vi "Project Data InitialS4.vi"(11 "configuration file path":path=path "C:/Users/MyUser/Desktop/新文字文件 - 複製.txt") -> (1 "Step Content":string[][](table), 2 "Retry":i32, 3 "process cluster":cluster{string[], i32[]})   [LabVIEW 2019]
uses:
  <vilib>/Utility/config.llb/Read Key (String).vi
  <vilib>/Utility/config.llb/NI_LVConfig.lvlib
  Ctrl/StationCmdSelect.ctl
  FlowCtrl Class/LineScan/LineScan.lvclass
  Ctrl/MeasureDisplayTab.ctl
  LLB/Commonly VI/Main Glb.vi
  LLB/Commonly VI.lvlib
  Ctrl/Table Save.ctl
  Ctrl/Auto Inspection Station Name2.ctl
  Ctrl/Auto Inspection Data Name.ctl
  Ctrl/S2 Station IO.ctl
panel:
  out "S2 receive":string
  out "Blue Scan2 receive":string
  out "T2 buffer":string
  out "T2 μA":dbl format="%#_6f"
  out "T1 buffer":string
  out "T1 μA":dbl format="%#_6f"
  in  "error in (no error)":errorcluster
  out "Blue Scan receive":string
  out "S1 receive":string
  out "Program receive":string
  out "Initial receive":string
  out "Act Step":i32
  out "retry次數":string[](array[string])
  in  "stop":bool
  out "Boolean":bool=TRUE
  in  "Numeric 3":i32
  out "format receive":string
  out "CurrentCmd":string
  out "Numeric":dbl
  out "LOG":string[][](array[string])
  in  "Enum":T1(ring)=enum."Add"
  in  "Table Control 3":string[][](table)=[["PCBA BARCODE", ""], ["硬體(Tool初始化)", ""], ["company(Tool初始化)", ""], ["耗電流 uA(電流表)", "T"], ["電池負載電壓", "T"], ["晶片ID(Tool FORMAT)", "F"], ["雷雕ID(TOOl scan、藍芽接收器)", "S"], ["Format(Tool FORMAT)", "F"], ["Programe(Tool Programe)", "P"]]
  in  "SN":string
  out "Array 3":cluster{"Table Control":string[][]}[](array[cluster])
  in  "Table Control":string[][](table)=[["PCBA BARCODE", ""], ["硬體(Tool初始化)", ""], ["company(Tool初始化)", ""], ["耗電流 uA(電流表)", "T"], ["電池負載電壓", "T"], ["晶片ID(Tool FORMAT)", "F"], ["雷雕ID(TOOl scan、藍芽接收器)", "S"], ["Format(Tool FORMAT)", "F"], ["Programe(Tool Programe)", "P"]]
  out "subarray":string[](array[string])
  out "array":string[](array[string])
  out "Process":string[](array[string])
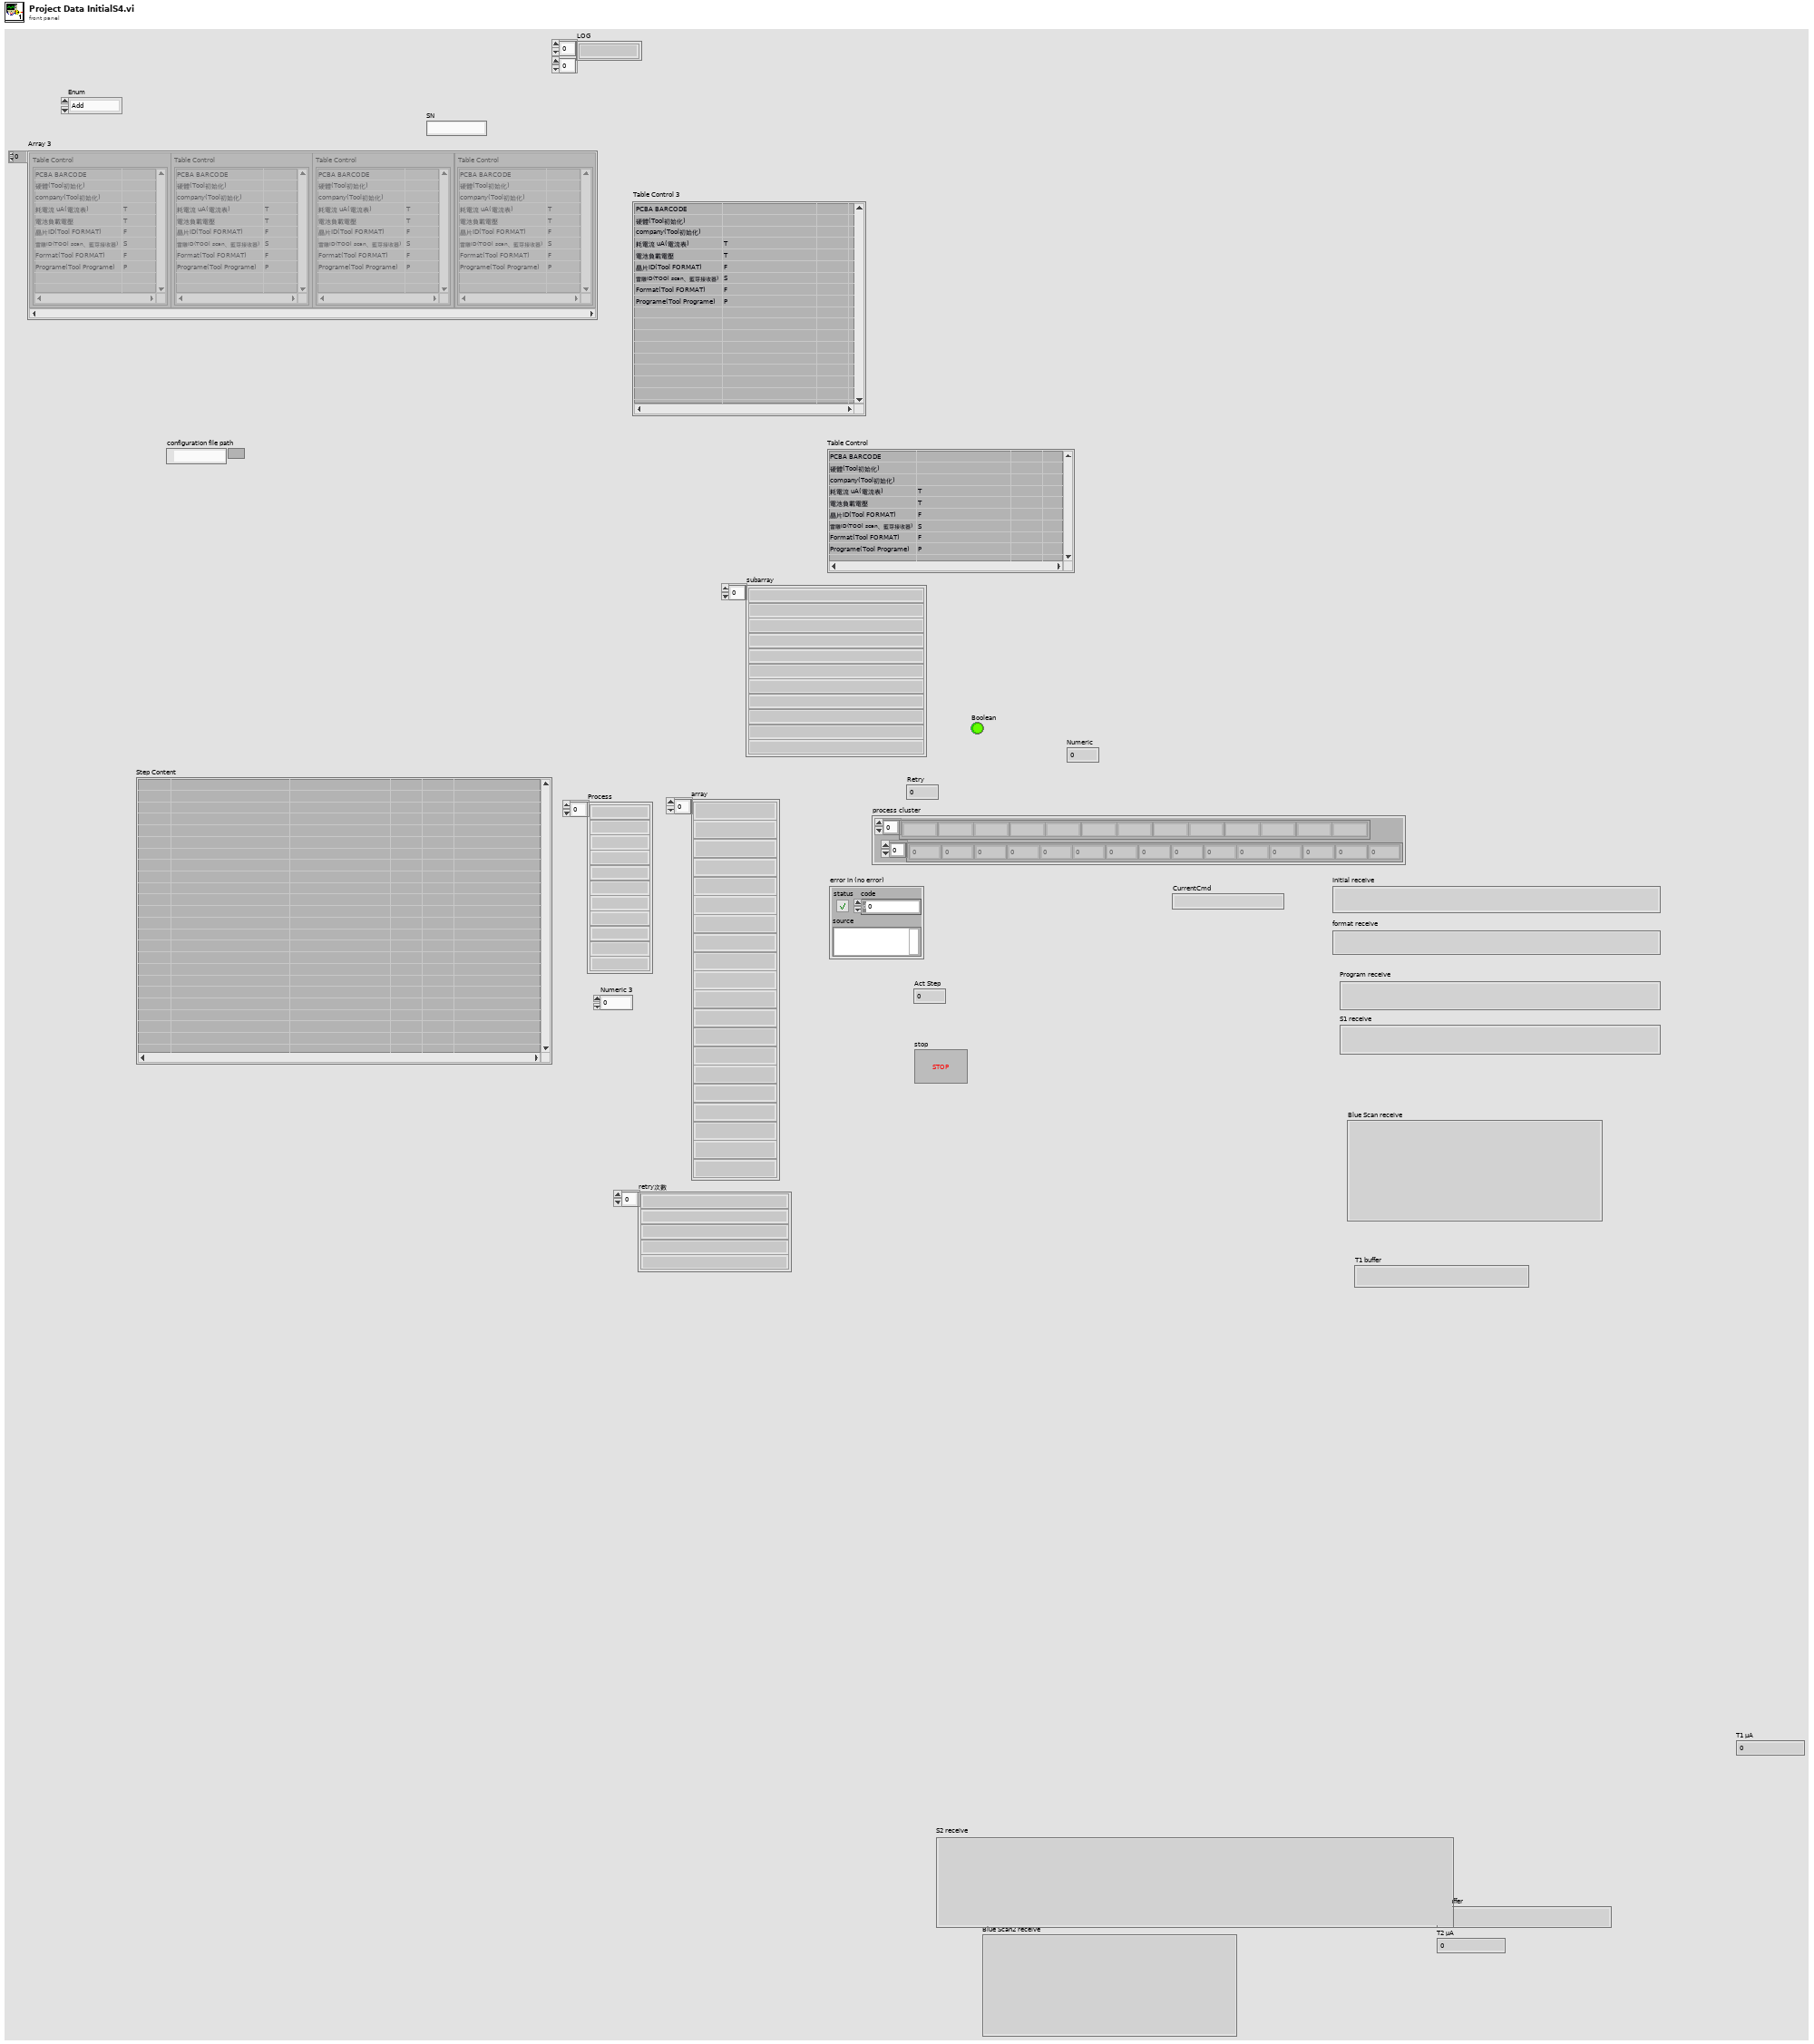
[diagram p1: front panel]
types:
  T1 = enum16{"initial", "Add", "Write", "Replace", "Delete", "REad"}
  T2 = typedef "NI_LVConfig.lvlib/Config Data RefNum.ctl" = refnum<k1>
  T3 = typedef "StationCmdSelect.ctl" = enum16{"Action", "Command", "Return", "DTime", "Retry"}
  T4 = typedef "Auto Inspection Data Name.ctl" = enum16{"LocalRun", "ItemSN(TimeCode)", "CurrentAction", "Error", "Data", "OKNG", "電壓值", "電壓值判斷", "電流值", "電流值判斷", "Laser1 Data", "Laser2 Data", "Laser OKNG", "StationNO"}
  T5 = typedef "Auto Inspection Station Name2.ctl" = enum16{"S1Barcode", "S2Measure", "S3Measure", "S4Measure", "S5Measure", "S11_LaserCheck", "S8_Vision AI"}
  T6 = typedef "Table Save.ctl" = enum16{"initial", "Add", "Write", "Replace", "Delete", "REad", "RedTable", "Load"}
  T7 = typedef "MeasureDisplayTab.ctl" = enum16{"Tray Barcode", "PCBA BARCODE", "硬體(Tool初始化)", "company(Tool初始化)", "耗電流 uA(電流表)", "電池負載電壓", "晶片ID(Tool FORMAT)", "雷雕ID(TOOl scan、藍芽接收器)", "Format(Tool FORMAT)", "Programe(Tool Programe)", "MAC(藍芽接收器)", "ID(藍芽接收器)", "KPA(藍芽接收器)", "溫度(藍芽接收器)", "SENSOR電池電壓(藍芽接收器)", "RSSI(藍芽接收器)", "SensorType_315(FSK scan)", "FSKsnVol_315(FSK scan)", "FSKscanl_315(FSK scan)", "P_315(FSK scan)", "T_315(FSK scan)", "SensorType_433(ASK scan)", "ASKsnVol_433(ASK scan)", "ASKscan_433(ASK scan)", "P_433(ASK scan)", "T_433(ASK scan)", "測高Data"}
  T8 = typedef "S2 Station IO.ctl" = enum16{"S2站PC動作中_20", "電流量測完成產品OK_21", "電流量測完成產品NG_22", "S2站Format 執行_23", "S2 Format OK_24", "S2 Format NG_25", "S2站燒入執行_26", "S2站燒入OK_27", "S2站燒入NG_28", "S2站動作完成_29", "S3 PC動作中_30", "S3 Format 此站執行_31", "S3 Format OK_32", "S3 Format NG_33", "S3 燒入程式 此站執行_34", "S3 燒入程式 OK_35", "S3 燒入程式 NG_36", "S3 備用_37", "S3 備用_38", "S3 動作完成_39", "S4 PC動作中_40", "S4 量測完成 產品正常_41", "S4 量測完成 產品NG_42", "S4 Format 此站執行_43", "S4 Format OK_44", "S4 Format NG_45", "S4 燒入 此站不執行_46", "S4 燒入程式 OK_47", "S4 燒入程式 NG_48", "S4 藍芽Scan OK_49", "S4 藍芽Scan NG_50", "S4 動作完成_51", "給PLC要量電流訊號", "給PLC要量電壓訊號"}
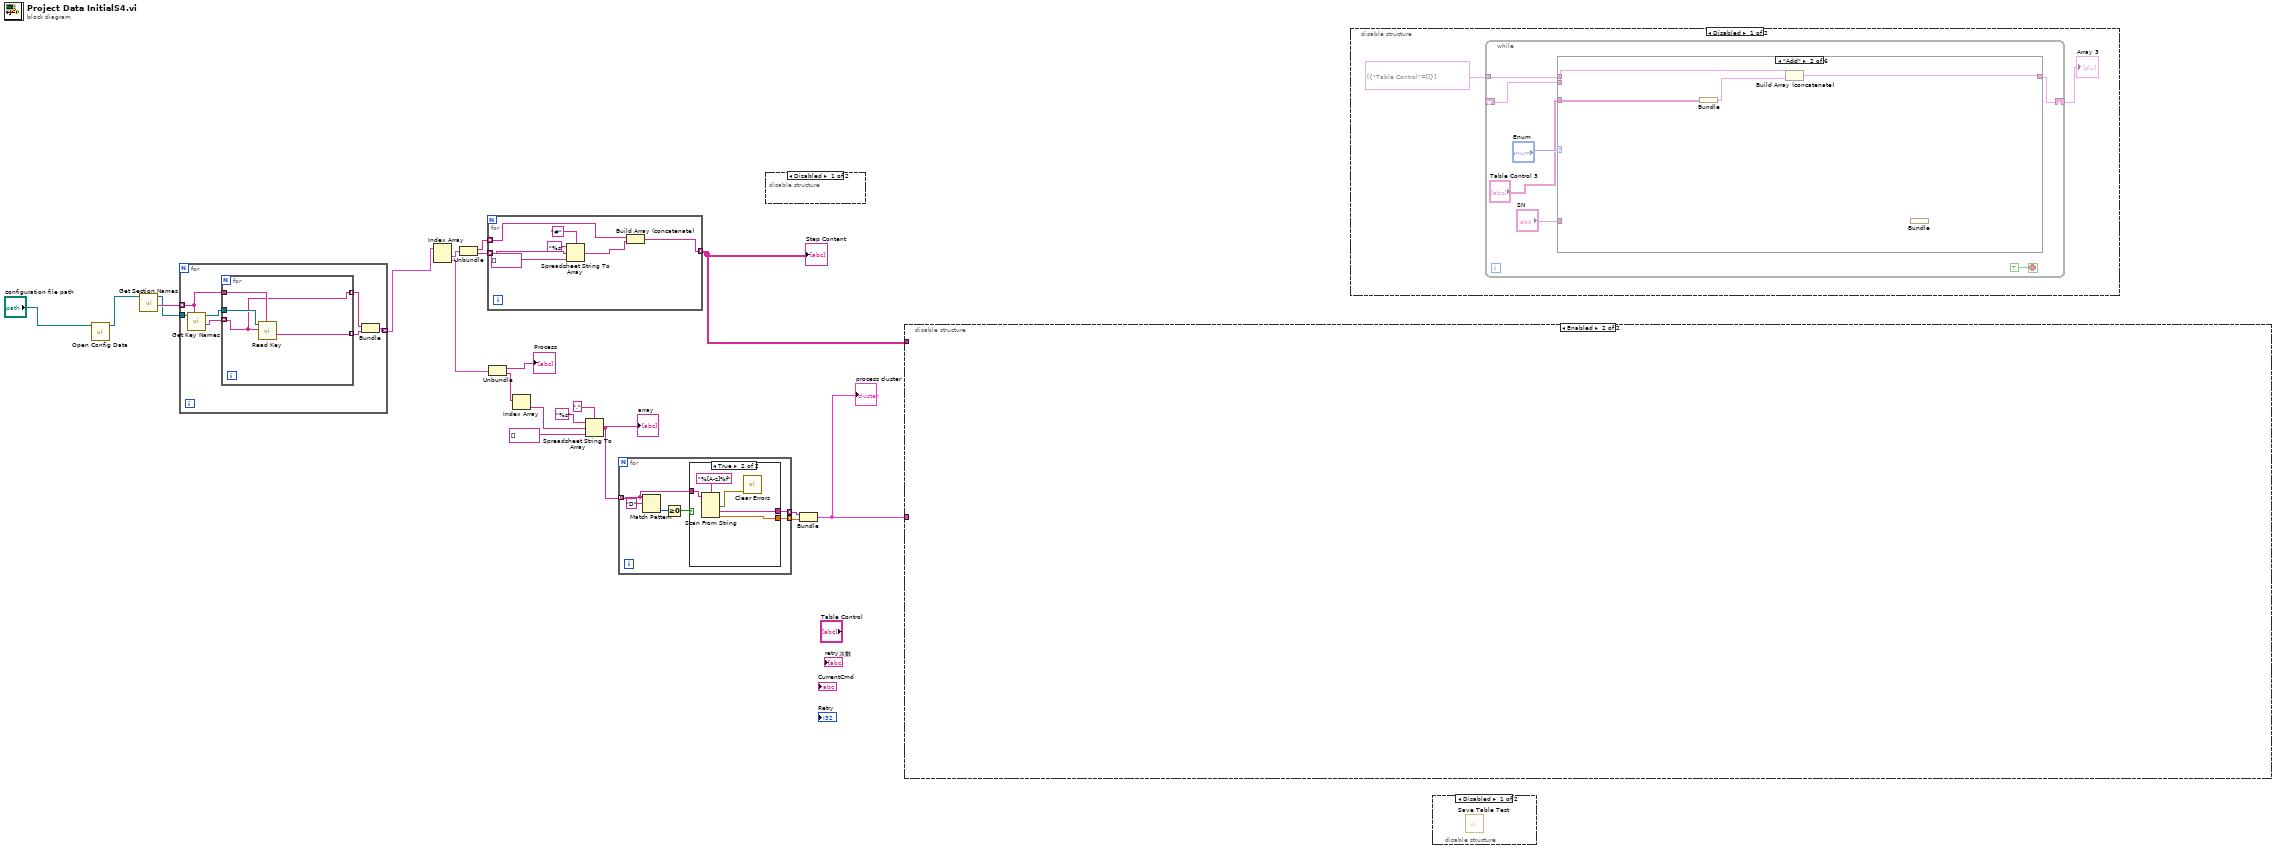
[diagram p0: block diagram]
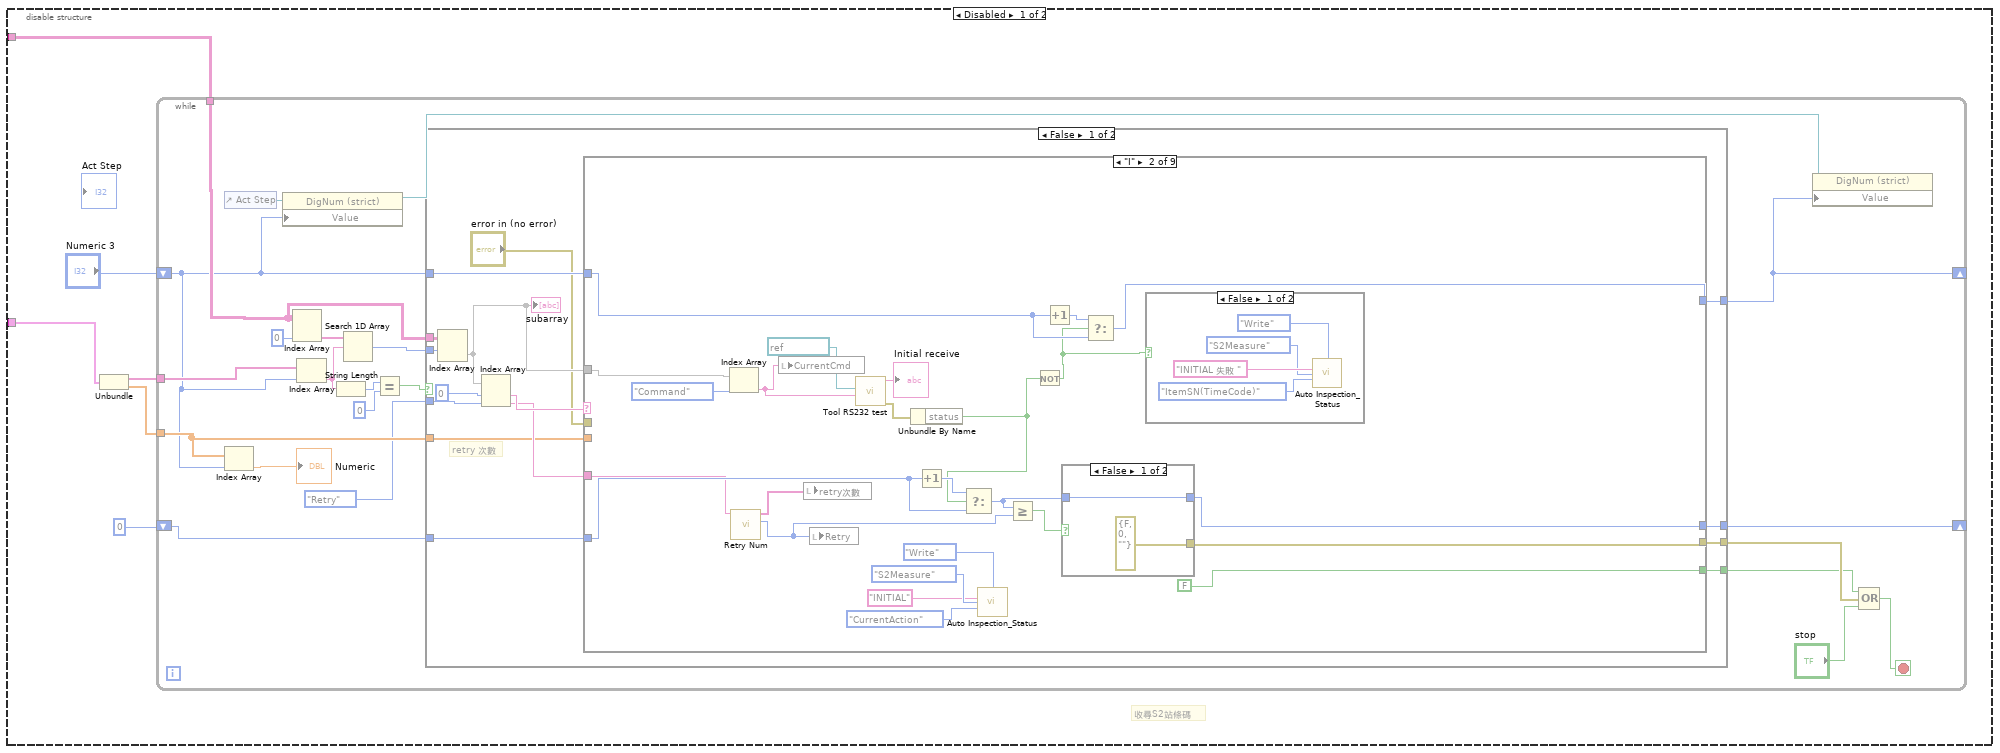
[diagram p3: hidden frame]
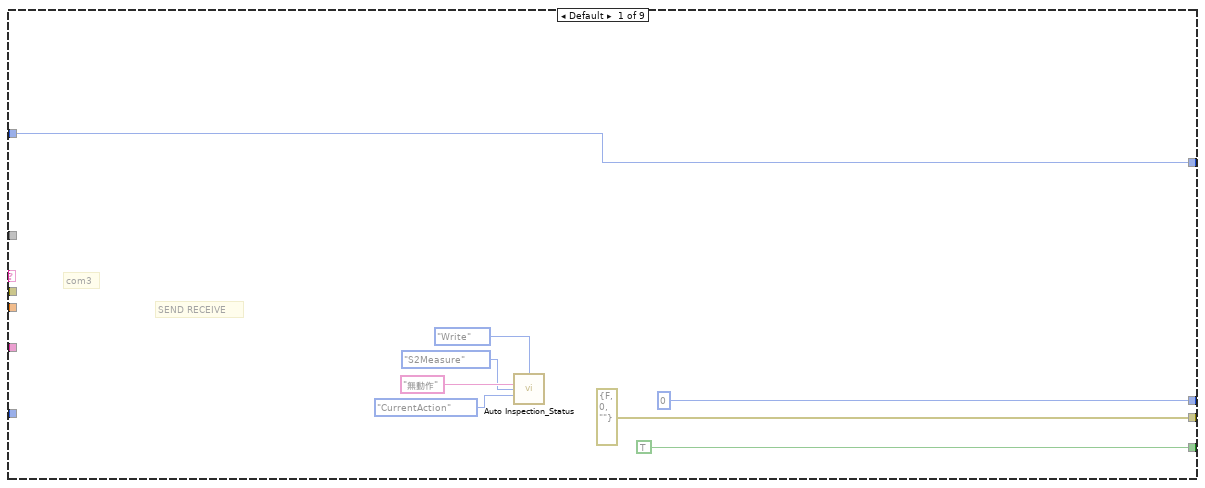
[diagram p4: hidden frame]
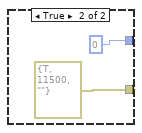
[diagram p6: hidden frame]
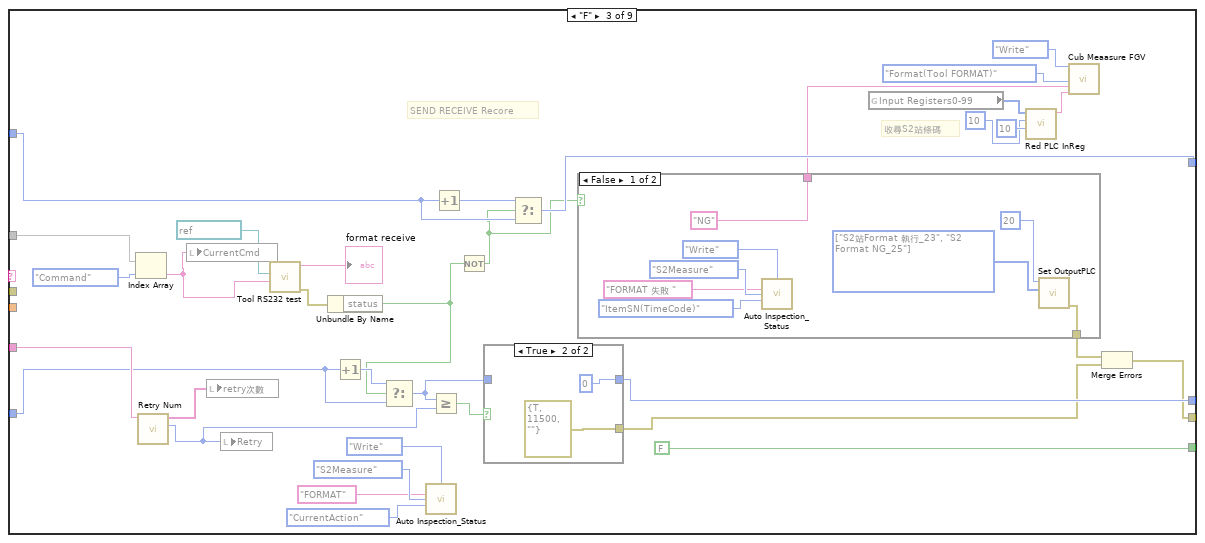
[diagram p7: hidden frame]
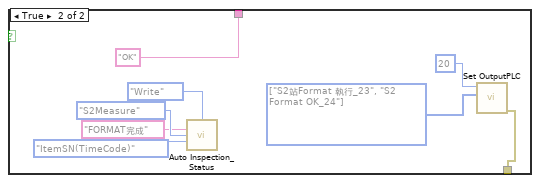
[diagram p8: hidden frame]
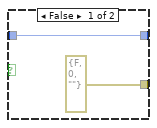
[diagram p9: hidden frame]
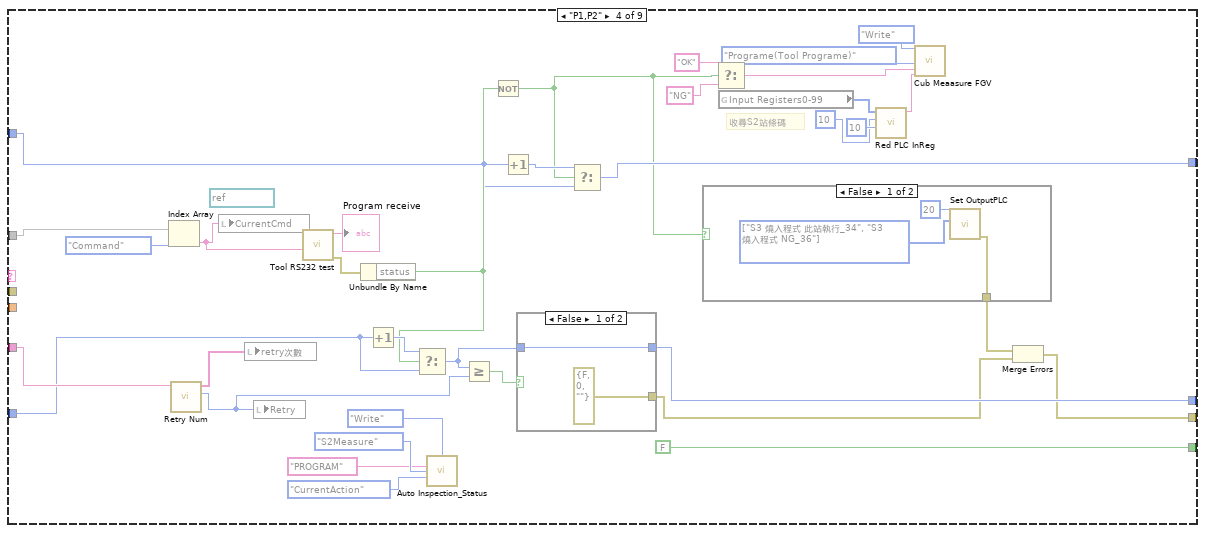
[diagram p10: hidden frame]
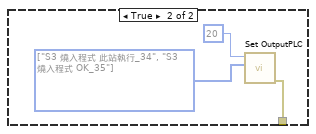
[diagram p11: hidden frame]
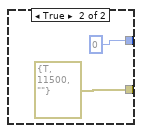
[diagram p12: hidden frame]
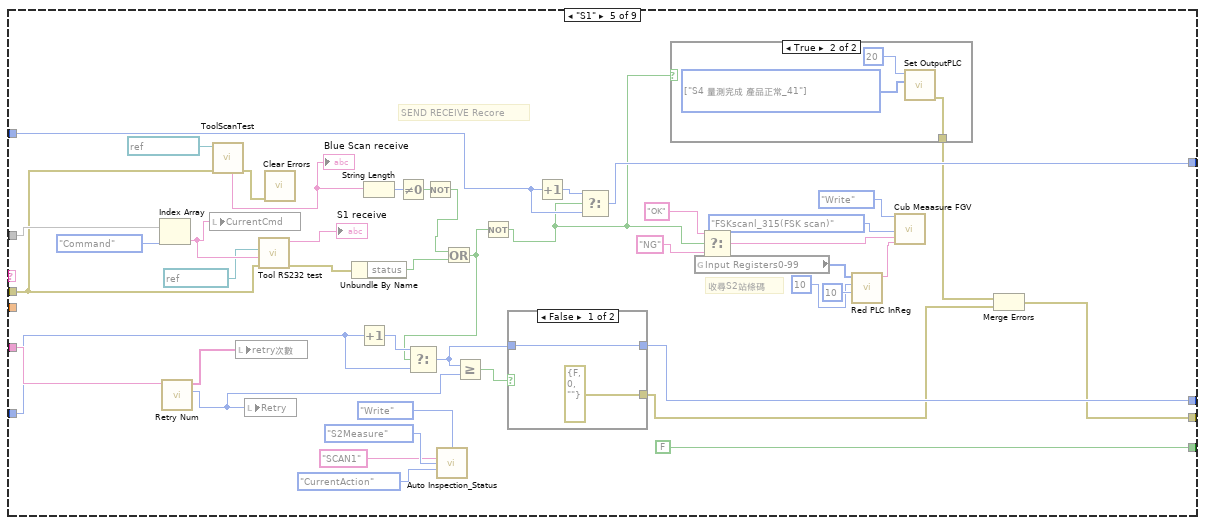
[diagram p13: hidden frame]
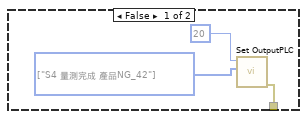
[diagram p14: hidden frame]
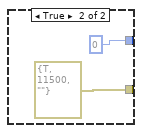
[diagram p15: hidden frame]
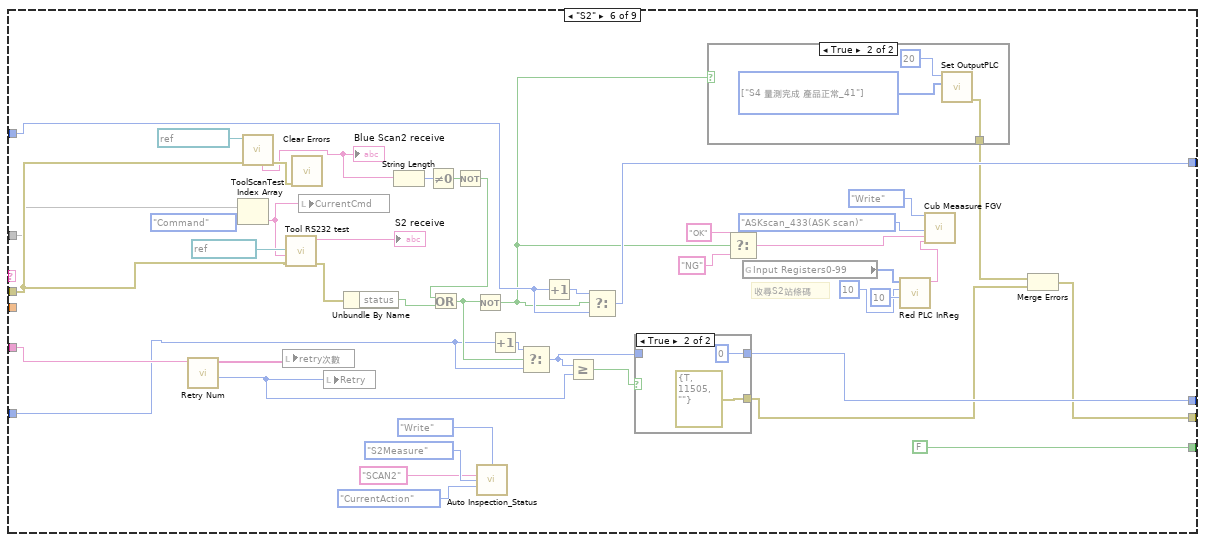
[diagram p16: hidden frame]
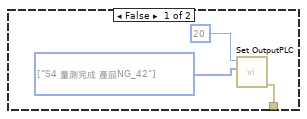
[diagram p17: hidden frame]
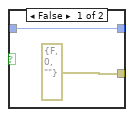
[diagram p18: hidden frame]
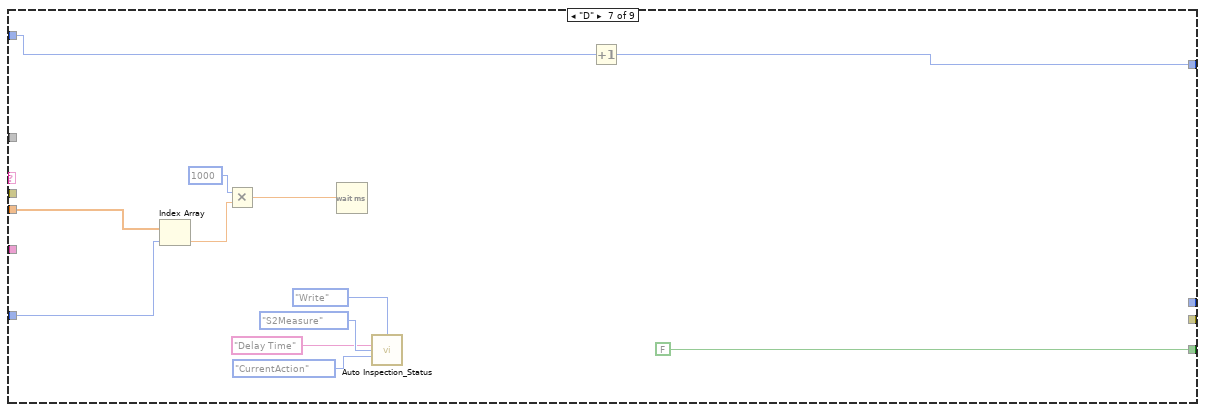
[diagram p19: hidden frame]
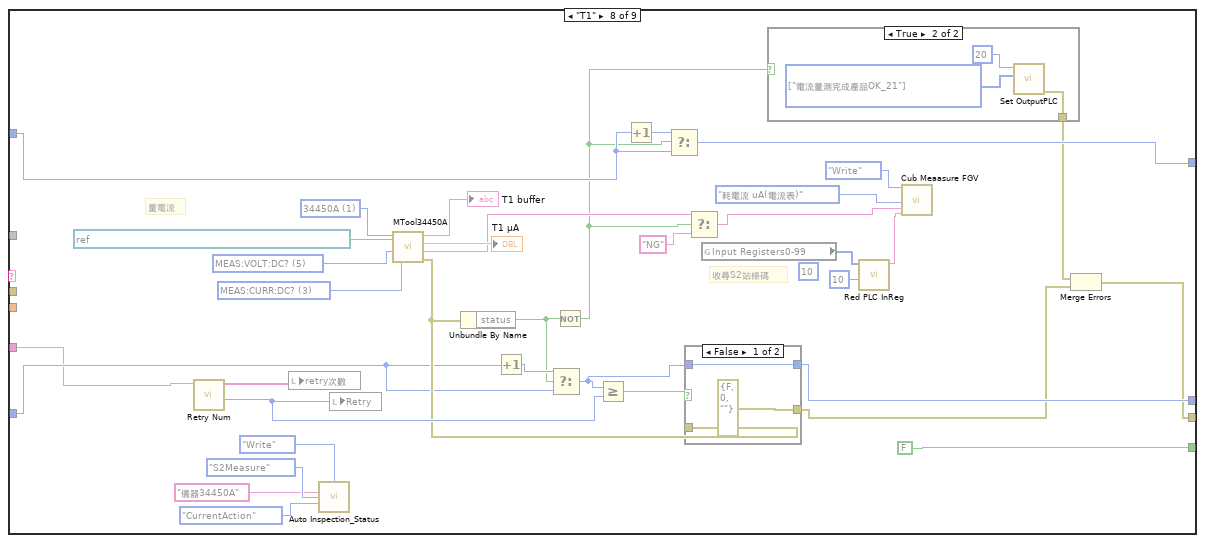
[diagram p20: hidden frame]
diagram:
  n1 = call <vilib>:"Open Config Data.vi"("configuration file path"="configuration file path") -> ("refnum"=w19:T2)  [unwired: 8 in, 2 out]
  n2 = call <vilib>:"Get Section Names.vi"("refnum"=w19) -> ("section names"=w18:string[], "refnum out"=w17:T2)  [unwired: 8 in, 1 out]
  n3 = for {
    tunnel: w17 -> [w27]
    tunnel: w18 -> [w22] mode=indexing
    tunnel: [w24] -> w15 mode=indexing
    n4 = call <vilib>:"Get Key Names.vi"("section"=w22, "refnum"=w27) -> ("key names"=w26:string[], "refnum out"=w23:T2)  [unwired: 6 in, 2 out]
    n5 = for {
      tunnel: w26 -> [w28] mode=indexing
      tunnel: [w31] -> w25 mode=indexing
      tunnel: w23 -> [w30]
      tunnel: w22 -> [w29]
      tunnel: [w28] -> w21 mode=indexing
      n6 = call-poly <vilib>:"Read Key.vi"("section"=w29, "key"=w28, "refnum"=w30) -> ("value"=w31:string)  [unwired: 5 in, 3 out]
    }
    n7 = Bundle(w21, w25) -> (w24:cluster{string[], string[]})  [unwired: 1 in]
  }
  n8 = Index Array(array=w15) -> (element #1=w11:cluster{string[], string[]}, element #2=w14:cluster{string[], string[]})  [unwired: 2 in]
  n9 = Unbundle(w11) -> (w12:string[], w13:string[])
  n10 = for {
    tunnel: w13 -> [w36] mode=indexing
    tunnel: [w32] -> w2 mode=indexing
    tunnel: w12 -> [w33] mode=indexing
    n11 = Spreadsheet String To Array(delimiter (Tab)="#", format string="%s", spreadsheet string=w36, array type (2D Dbl)=string[] []) -> (array=w34:string[])
    n12 = Build Array (concatenate)(w33, w34) -> (w32:string[])
  }
  "Step Content" <- w2
  n13 = Unbundle(w14) -> (→"Process":string[], w7:string[])
  n14 = Index Array(array=w7) -> (element=w6:string)  [unwired: 1 in]
  n15 = Spreadsheet String To Array(delimiter (Tab)=",", format string="%s", spreadsheet string=w6, array type (2D Dbl)=string[] []) -> (array=w5:string[])
  "array" <- w5
  n16 = for {
    tunnel: w5 -> [w39] mode=indexing
    tunnel: [w44] -> w4 mode=indexing
    tunnel: [w43] -> w3 mode=indexing
    n17 = Match Pattern(string=w39, regular expression="D") -> (offset past match=w41:i32)  [unwired: 1 in, 3 out]
    n18 = Greater Or Equal To 0?(x=w41) -> (x >= 0?=w40:bool)
    n19 = case shown="True" w40 {
      tunnel: [w46 w50] -> w44
      tunnel: [-1.0 w49] -> w43
      tunnel: w39 -> [w46 w47]
      frame False {
      }
      frame True {
        n20 = Scan From String(format string="%[A-z]%f", input string=w47) -> (error out=w48:errorcluster, output 1=w50:string, output 2=w49:dbl)  [unwired: 4 in, 2 out]
        n21 = call <vilib>:"Clear Errors.vi"("error in (no error)"=w48) -> ()  [unwired: 5 in, 2 out]
      }
    }
  }
  n22 = disable-structure shown="Disabled" {
    frame Disabled {
    }
    frame Enabled {
    }
  }
  n23 = Bundle(w4, w3) -> (w1:cluster{string[], dbl[]})  [unwired: 1 in]
  "process cluster" <- w1
  n24 = disable-structure shown="Enabled" {
    disable-tunnel: w2 -> [w55 _]
    disable-tunnel: w1 -> [w54 _]
    frame Disabled {
      # "收尋S2站條碼"
      n25 = Unbundle(w54) -> (w57:string[], w56:dbl[])
      n26 = while {
        tunnel: w57 -> [w79]
        tunnel: w56 -> [w78]
        tunnel: w55 -> [w77]
        shift-right: [w60] -> _
        shift-left: 0 -> [w64]
        shift-right: [w61] -> _
        shift-left: "Numeric 3" -> [w58]
        stop <- w65 stop-if-true
        n27 = control-ref of="Act Step"() -> (w63:refnum<vi>)
        n28 = Index Array(array=w78, index=w58) -> (element=→"Numeric":dbl)
        n29 = property class="DigNum (strict)"(reference=w63, "Value"=w58) -> (reference out=w62:refnum<vi>)  [unwired: 1 in, 1 out]
        n30 = Index Array(array=w77, index (col)=0 ("disabled index (col)")) -> (element=w75:string[])  [unwired: 1 in]
        n31 = Index Array(array=w79, index=w58) -> (element=w72:string)
        n32 = String Length(string=w72) -> (length=w71:i32)
        n33 = Search 1D Array(1D array=w75, element=w72) -> (index of element=w74:i32)  [unwired: 1 in]
        n34 = Equal?(x=w71, y=0) -> (x = y?=w69:bool)
        n35 = case shown="False" w69 {
          tunnel: w77 -> [w94 _]
          tunnel: w74 -> [w93 _]
          tunnel: w78 -> [w89 _]
          tunnel: w64 -> [w87 _]
          tunnel: StationCmdSelect."Retry" -> [w86 _]
          tunnel: [w85 _] -> w66
          tunnel: w58 -> [w84 _]
          tunnel: [w83 _] -> w61
          tunnel: [w82 _] -> w60
          tunnel: [w81 w447] -> w59
          frame False {
            # "retry 次數"
            n36 = Index Array(array=w94, index (row)=w93) -> (element=w88:string[])  [unwired: 1 in]
            "subarray" <- w88
            n37 = Index Array(array=w88, index #1=0 ("index"), index #2=w86) -> (element #1=w91:string, element #2=w90:string)
            n38 = case shown="\"I\"" w91 {
              tunnel: w89 -> [_ _ _ _ _ _ w353 _ _]
              tunnel: w90 -> [_ w112 w165 w211 w267 w312 _ w374 w419]
              tunnel: w88 -> [_ w114 w169 w210 w264 w313 _ _ _]
              tunnel: w87 -> [_ w113 w162 w208 w261 w311 w350 w375 w420]
              tunnel: [errorcluster {"status"=FALSE, "code"=0, "source"=""} ("error constant") w117 w136 w190 w235 w289 _ w355 w401] -> w85
              tunnel: w84 -> [w102 w115 w157 w207 w266 w315 w348 w373 w421]
              tunnel: [w102 w111 w156 w213 w265 w308 w347 w372 w422] -> w83
              tunnel: [0 w116 w154 w212 w268 w310 _ w371 w424] -> w82
              tunnel: [TRUE FALSE FALSE FALSE FALSE FALSE FALSE FALSE FALSE] -> w81
              tunnel: "error in (no error)" -> [_ _ _ _ w258 w314 _ _ _]
              frame Default {
                # "SEND RECEIVE"
                # "com3"
                n39 = call "Auto Inspection_Status.vi"("Action"=enum16{"Initial", "Write", "Read"}."Write", "DataIn"="無動作", "Station"=Auto_Inspection_Station_Name2."S2Measure", "Data"=Auto_Inspection_Data_Name."CurrentAction") -> ()  [unwired: 9 in, 3 out]
              }
              frame "I" {
                n40 = Index Array(array=w114, index=StationCmdSelect."Command") -> (element=w109:string)
                n41 = call "Retry Num.vi"("String"=w112) -> ("Numeric"=w124:i32, "retry次數"=w110:string[])  [unwired: 9 in]
                n42 = local write "CurrentCmd"(w109) -> ()
                n43 = local write "retry次數"(w110) -> ()
                n44 = local write "Retry"(w124) -> ()
                n45 = call "Tool RS232 test.vi"("Cmd In"=w109, "VISA resource name"=refnum<visa-resource-name> "COM8") -> ("error out"=w125:errorcluster, "receive string"=→"Initial receive":string)  [unwired: 8 in]
                n46 = Unbundle By Name(w125) -> ("status"=w121:bool)
                n47 = Increment(x=w113) -> (x+1=w126:i32)
                n48 = Select(t=w126, s=w121, f=w113) -> (s? t:f=w120:i32)
                n49 = call "Auto Inspection_Status.vi"("Action"=enum16{"Initial", "Write", "Read"}."Write", "DataIn"="INITIAL", "Station"=Auto_Inspection_Station_Name2."S2Measure", "Data"=Auto_Inspection_Data_Name."CurrentAction") -> ()  [unwired: 9 in, 3 out]
                n50 = Greater Or Equal?(x=w120, y=w124) -> (x >= y?=w123:bool)
                n51 = Not(x=w121) -> (.not. x?=w103:bool)
                n52 = Increment(x=w115) -> (x+1=w122:i32)
                n53 = case shown="False" w123 {
                  tunnel: [errorcluster {"status"=FALSE, "code"=0, "source"=""} ("error constant") errorcluster {"status"=TRUE, "code"=11500, "source"=""} ("error constant")] -> w117
                  tunnel: w120 -> [w132 _]
                  tunnel: [w132 0] -> w116
                  frame False {
                  }
                  frame True {
                  }
                }
                n54 = Select(t=w122, s=w103, f=w115) -> (s? t:f=w111:i32)
                n55 = case shown="False" w103 {
                  frame False {
                    n56 = call "Auto Inspection_Status.vi"("Action"=enum16{"Initial", "Write", "Read"}."Write", "DataIn"="INITIAL 失敗 ", "Station"=Auto_Inspection_Station_Name2."S2Measure", "Data"=Auto_Inspection_Data_Name."ItemSN(TimeCode)") -> ()  [unwired: 9 in, 3 out]
                  }
                  frame True {
                  }
                }
              }
              frame "F" {
                # "收尋S2站條碼"
                # "SEND RECEIVE Recore"
                n57 = Index Array(array=w169, index=StationCmdSelect."Command") -> (element=w153:string)
                n58 = call "Retry Num.vi"("String"=w165) -> ("Numeric"=w161:i32, "retry次數"=w152:string[])  [unwired: 9 in]
                n59 = local write "CurrentCmd"(w153) -> ()
                n60 = local write "retry次數"(w152) -> ()
                n61 = local write "Retry"(w161) -> ()
                n62 = call "Tool RS232 test.vi"("Cmd In"=w153, "VISA resource name"=refnum<visa-resource-name> "COM8") -> ("error out"=w163:errorcluster, "receive string"=→"format receive":string)  [unwired: 8 in]
                n63 = Unbundle By Name(w163) -> ("status"=w158:bool)
                n64 = Increment(x=w162) -> (x+1=w164:i32)
                n65 = Select(t=w164, s=w158, f=w162) -> (s? t:f=w155:i32)
                n66 = call "Auto Inspection_Status.vi"("Action"=enum16{"Initial", "Write", "Read"}."Write", "DataIn"="FORMAT", "Station"=Auto_Inspection_Station_Name2."S2Measure", "Data"=Auto_Inspection_Data_Name."CurrentAction") -> ()  [unwired: 9 in, 3 out]
                n67 = Greater Or Equal?(x=w155, y=w161) -> (x >= y?=w160:bool)
                n68 = Increment(x=w157) -> (x+1=w159:i32)
                n69 = Not(x=w158) -> (.not. x?=w150:bool)
                n70 = case shown="True" w160 {
                  tunnel: [errorcluster {"status"=FALSE, "code"=0, "source"=""} ("error constant") errorcluster {"status"=TRUE, "code"=11500, "source"=""} ("error constant")] -> w137
                  tunnel: w155 -> [w186 _]
                  tunnel: [w186 0] -> w154
                  frame False {
                  }
                  frame True {
                  }
                }
                n71 = Select(t=w159, s=w150, f=w157) -> (s? t:f=w156:i32)
                n72 = case shown="False" w150 {
                  tunnel: ["NG" "OK"] -> w143
                  tunnel: [w170 w178] -> w138
                  frame False {
                    w172 = T8[] [enum."S2站Format 執行_23", enum."S2 Format NG_25"] items=["S2站PC動作中_20", "電流量測完成產品OK_21", "電流量測完成產品NG_22", "S2站Format 執行_23", "S2 Format OK_24", "S2 Format NG_25", "S2站燒入執行_26", "S2站燒入OK_27", "S2站燒入NG_28", "S2站動作完成_29", "S3 PC動作中_30", "S3 Format 此站執行_31", "S3 Format OK_32", "S3 Format NG_33", "S3 燒入程式 此站執行_34", "S3 燒入程式 OK_35", "S3 燒入程式 NG_36", "S3 備用_37", "S3 備用_38", "S3 動作完成_39", "S4 PC動作中_40", "S4 量測完成 產品正常_41", "S4 量測完成 產品NG_42", "S4 Format 此站執行_43", "S4 Format OK_44", "S4 Format NG_45", "S4 燒入 此站不執行_46", "S4 燒入程式 OK_47", "S4 燒入程式 NG_48", "S4 藍芽Scan OK_49", "S4 藍芽Scan NG_50", "S4 動作完成_51", "給PLC要量電流訊號", "給PLC要量電壓訊號"]
                    n73 = call "Auto Inspection_Status.vi"("Action"=enum16{"Initial", "Write", "Read"}."Write", "DataIn"="FORMAT 失敗 ", "Station"=Auto_Inspection_Station_Name2."S2Measure", "Data"=Auto_Inspection_Data_Name."ItemSN(TimeCode)") -> ()  [unwired: 9 in, 3 out]
                    n74 = call "Set OutputPLC.vi"("Address In"=20, "Array 2"=w172) -> ("Error Out"=w170:errorcluster[])  [unwired: 8 in]
                  }
                  frame True {
                    w180 = T8[] [enum."S2站Format 執行_23", enum."S2 Format OK_24"] items=["S2站PC動作中_20", "電流量測完成產品OK_21", "電流量測完成產品NG_22", "S2站Format 執行_23", "S2 Format OK_24", "S2 Format NG_25", "S2站燒入執行_26", "S2站燒入OK_27", "S2站燒入NG_28", "S2站動作完成_29", "S3 PC動作中_30", "S3 Format 此站執行_31", "S3 Format OK_32", "S3 Format NG_33", "S3 燒入程式 此站執行_34", "S3 燒入程式 OK_35", "S3 燒入程式 NG_36", "S3 備用_37", "S3 備用_38", "S3 動作完成_39", "S4 PC動作中_40", "S4 量測完成 產品正常_41", "S4 量測完成 產品NG_42", "S4 Format 此站執行_43", "S4 Format OK_44", "S4 Format NG_45", "S4 燒入 此站不執行_46", "S4 燒入程式 OK_47", "S4 燒入程式 NG_48", "S4 藍芽Scan OK_49", "S4 藍芽Scan NG_50", "S4 動作完成_51", "給PLC要量電流訊號", "給PLC要量電壓訊號"]
                    n75 = call "Auto Inspection_Status.vi"("Action"=enum16{"Initial", "Write", "Read"}."Write", "DataIn"="FORMAT完成", "Station"=Auto_Inspection_Station_Name2."S2Measure", "Data"=Auto_Inspection_Data_Name."ItemSN(TimeCode)") -> ()  [unwired: 9 in, 3 out]
                    n76 = call "Set OutputPLC.vi"("Address In"=20, "Array 2"=w180) -> ("Error Out"=w178:errorcluster[])  [unwired: 8 in]
                  }
                }
                n77 = global read "Main Glb.vi" "Input Registers0-99"() -> (w142:u16[])
                n78 = call "Red PLC InReg.vi"("length"=10, "index"=10, "Input Registers Arr"=w142) -> ("Rad In Reg"=w139:string)  [unwired: 7 in, 1 out]
                n79 = call "Cub Meaasure FGV.vi"("Action"=Table_Save."Write" ("Enum"), "Save Index"=MeasureDisplayTab."Format(Tool FORMAT)", "DataIn"=w143, "SN"=w139) -> ()  [unwired: 8 in, 8 out]
                n80 = Merge Errors(w138, w137) -> (w136:errorcluster)
              }
              frame "P1,P2" {
                (unwired) refnum<visa-resource-name> "COM8" ("VISA resource name")
                # "收尋S2站條碼"
                n81 = Index Array(array=w210, index=StationCmdSelect."Command") -> (element=w224:string)
                n82 = call "Retry Num.vi"("String"=w211) -> ("Numeric"=w219:i32, "retry次數"=w223:string[])  [unwired: 9 in]
                n83 = local write "CurrentCmd"(w224) -> ()
                n84 = local write "retry次數"(w223) -> ()
                n85 = local write "Retry"(w219) -> ()
                n86 = call "Tool RS232 test.vi"("Cmd In"=w224) -> ("error out"=w220:errorcluster, "receive string"=→"Program receive":string)  [unwired: 9 in]
                n87 = Unbundle By Name(w220) -> ("status"=w216:bool)
                n88 = Increment(x=w208) -> (x+1=w221:i32)
                n89 = Select(t=w221, s=w216, f=w208) -> (s? t:f=w215:i32)
                n90 = call "Auto Inspection_Status.vi"("Action"=enum16{"Initial", "Write", "Read"}."Write", "DataIn"="PROGRAM", "Station"=Auto_Inspection_Station_Name2."S2Measure", "Data"=Auto_Inspection_Data_Name."CurrentAction") -> ()  [unwired: 9 in, 3 out]
                n91 = Greater Or Equal?(x=w215, y=w219) -> (x >= y?=w218:bool)
                n92 = Not(x=w216) -> (.not. x?=w193:bool)
                n93 = Increment(x=w207) -> (x+1=w217:i32)
                n94 = case shown="False" w218 {
                  tunnel: [errorcluster {"status"=FALSE, "code"=0, "source"=""} ("error constant") errorcluster {"status"=TRUE, "code"=11500, "source"=""} ("error constant")] -> w192
                  tunnel: w215 -> [w231 _]
                  tunnel: [w231 0] -> w212
                  frame False {
                  }
                  frame True {
                  }
                }
                n95 = Select(t=w217, s=w193, f=w207) -> (s? t:f=w213:i32)
                n96 = case shown="False" w193 {
                  tunnel: [w225 w228] -> w191
                  frame False {
                    w227 = T8[] [enum."S3 燒入程式 此站執行_34", enum."S3 燒入程式 NG_36"] items=["S2站PC動作中_20", "電流量測完成產品OK_21", "電流量測完成產品NG_22", "S2站Format 執行_23", "S2 Format OK_24", "S2 Format NG_25", "S2站燒入執行_26", "S2站燒入OK_27", "S2站燒入NG_28", "S2站動作完成_29", "S3 PC動作中_30", "S3 Format 此站執行_31", "S3 Format OK_32", "S3 Format NG_33", "S3 燒入程式 此站執行_34", "S3 燒入程式 OK_35", "S3 燒入程式 NG_36", "S3 備用_37", "S3 備用_38", "S3 動作完成_39", "S4 PC動作中_40", "S4 量測完成 產品正常_41", "S4 量測完成 產品NG_42", "S4 Format 此站執行_43", "S4 Format OK_44", "S4 Format NG_45", "S4 燒入 此站不執行_46", "S4 燒入程式 OK_47", "S4 燒入程式 NG_48", "S4 藍芽Scan OK_49", "S4 藍芽Scan NG_50", "S4 動作完成_51", "給PLC要量電流訊號", "給PLC要量電壓訊號"]
                    n97 = call "Set OutputPLC.vi"("Address In"=20, "Array 2"=w227) -> ("Error Out"=w225:errorcluster[])  [unwired: 8 in]
                  }
                  frame True {
                    w229 = T8[] [enum."S3 燒入程式 此站執行_34", enum."S3 燒入程式 OK_35"] items=["S2站PC動作中_20", "電流量測完成產品OK_21", "電流量測完成產品NG_22", "S2站Format 執行_23", "S2 Format OK_24", "S2 Format NG_25", "S2站燒入執行_26", "S2站燒入OK_27", "S2站燒入NG_28", "S2站動作完成_29", "S3 PC動作中_30", "S3 Format 此站執行_31", "S3 Format OK_32", "S3 Format NG_33", "S3 燒入程式 此站執行_34", "S3 燒入程式 OK_35", "S3 燒入程式 NG_36", "S3 備用_37", "S3 備用_38", "S3 動作完成_39", "S4 PC動作中_40", "S4 量測完成 產品正常_41", "S4 量測完成 產品NG_42", "S4 Format 此站執行_43", "S4 Format OK_44", "S4 Format NG_45", "S4 燒入 此站不執行_46", "S4 燒入程式 OK_47", "S4 燒入程式 NG_48", "S4 藍芽Scan OK_49", "S4 藍芽Scan NG_50", "S4 動作完成_51", "給PLC要量電流訊號", "給PLC要量電壓訊號"]
                    n98 = call "Set OutputPLC.vi"("Address In"=20, "Array 2"=w229) -> ("Error Out"=w228:errorcluster[])  [unwired: 8 in]
                  }
                }
                n99 = Select(t="OK" ("DataIn"), s=w193, f="NG" ("DataIn")) -> (s? t:f=w194:string)
                n100 = global read "Main Glb.vi" "Input Registers0-99"() -> (w202:u16[])
                n101 = call "Red PLC InReg.vi"("length"=10, "index"=10, "Input Registers Arr"=w202) -> ("Rad In Reg"=w201:string)  [unwired: 7 in, 1 out]
                n102 = call "Cub Meaasure FGV.vi"("Action"=Table_Save."Write" ("Enum"), "Save Index"=MeasureDisplayTab."Programe(Tool Programe)", "DataIn"=w194, "SN"=w201) -> ()  [unwired: 8 in, 8 out]
                n103 = Merge Errors(w191, w192) -> (w190:errorcluster)
              }
              frame "S1" {
                # "收尋S2站條碼"
                # "SEND RECEIVE Recore"
                n104 = Index Array(array=w264, index=StationCmdSelect."Command") -> (element=w277:string)
                n105 = call "Retry Num.vi"("String"=w267) -> ("Numeric"=w272:i32, "retry次數"=w276:string[])  [unwired: 9 in]
                n106 = local write "CurrentCmd"(w277) -> ()
                n107 = call "ToolScanTest.vi"("error in (no error)"=w258, "VISA resource name"=refnum<visa-resource-name> "COM10") -> ("error out"=w259:errorcluster, "read string 6"=w255:string)  [unwired: 4 in, 4 out]
                "Blue Scan receive" <- w255
                n108 = local write "retry次數"(w276) -> ()
                n109 = local write "Retry"(w272) -> ()
                n110 = call "Tool RS232 test.vi"("error in (no error)"=w258, "Cmd In"=w277, "VISA resource name"=refnum<visa-resource-name> "COM8") -> ("error out"=w273:errorcluster, "receive string"=→"S1 receive":string)  [unwired: 7 in]
                n111 = call <vilib>:"Clear Errors.vi"("error in (no error)"=w259) -> ()  [unwired: 5 in, 2 out]
                n112 = Unbundle By Name(w273) -> ("status"=w253:bool)
                n113 = Increment(x=w261) -> (x+1=w274:i32)
                n114 = String Length(string=w255) -> (length=w257:i32)
                n115 = Not Equal To 0?(x=w257) -> (x != 0?=w256:bool)
                n116 = Not(x=w256) -> (.not. x?=w254:bool)
                n117 = call "Auto Inspection_Status.vi"("Action"=enum16{"Initial", "Write", "Read"}."Write", "DataIn"="SCAN1", "Station"=Auto_Inspection_Station_Name2."S2Measure", "Data"=Auto_Inspection_Data_Name."CurrentAction") -> ()  [unwired: 9 in, 3 out]
                n118 = Or(x=w254, y=w253) -> (x .or. y?=w252:bool)
                n119 = Select(t=w274, s=w252, f=w261) -> (s? t:f=w269:i32)
                n120 = Greater Or Equal?(x=w269, y=w272) -> (x >= y?=w271:bool)
                n121 = Not(x=w252) -> (.not. x?=w238:bool)
                n122 = case shown="False" w271 {
                  tunnel: [errorcluster {"status"=FALSE, "code"=0, "source"=""} ("error constant") errorcluster {"status"=TRUE, "code"=11500, "source"=""} ("error constant")] -> w236
                  tunnel: w269 -> [w285 _]
                  tunnel: [w285 0] -> w268
                  frame False {
                  }
                  frame True {
                  }
                }
                n123 = Increment(x=w266) -> (x+1=w270:i32)
                n124 = Select(t=w270, s=w238, f=w266) -> (s? t:f=w265:i32)
                n125 = case shown="True" w238 {
                  tunnel: [w279 w283] -> w237
                  frame False {
                    w281 = T8[] [enum."S4 量測完成 產品NG_42"] items=["S2站PC動作中_20", "電流量測完成產品OK_21", "電流量測完成產品NG_22", "S2站Format 執行_23", "S2 Format OK_24", "S2 Format NG_25", "S2站燒入執行_26", "S2站燒入OK_27", "S2站燒入NG_28", "S2站動作完成_29", "S3 PC動作中_30", "S3 Format 此站執行_31", "S3 Format OK_32", "S3 Format NG_33", "S3 燒入程式 此站執行_34", "S3 燒入程式 OK_35", "S3 燒入程式 NG_36", "S3 備用_37", "S3 備用_38", "S3 動作完成_39", "S4 PC動作中_40", "S4 量測完成 產品正常_41", "S4 量測完成 產品NG_42", "S4 Format 此站執行_43", "S4 Format OK_44", "S4 Format NG_45", "S4 燒入 此站不執行_46", "S4 燒入程式 OK_47", "S4 燒入程式 NG_48", "S4 藍芽Scan OK_49", "S4 藍芽Scan NG_50", "S4 動作完成_51", "給PLC要量電流訊號", "給PLC要量電壓訊號"]
                    n126 = call "Set OutputPLC.vi"("Address In"=20, "Array 2"=w281) -> ("Error Out"=w279:errorcluster[])  [unwired: 8 in]
                  }
                  frame True {
                    w282 = T8[] [enum."S4 量測完成 產品正常_41"] items=["S2站PC動作中_20", "電流量測完成產品OK_21", "電流量測完成產品NG_22", "S2站Format 執行_23", "S2 Format OK_24", "S2 Format NG_25", "S2站燒入執行_26", "S2站燒入OK_27", "S2站燒入NG_28", "S2站動作完成_29", "S3 PC動作中_30", "S3 Format 此站執行_31", "S3 Format OK_32", "S3 Format NG_33", "S3 燒入程式 此站執行_34", "S3 燒入程式 OK_35", "S3 燒入程式 NG_36", "S3 備用_37", "S3 備用_38", "S3 動作完成_39", "S4 PC動作中_40", "S4 量測完成 產品正常_41", "S4 量測完成 產品NG_42", "S4 Format 此站執行_43", "S4 Format OK_44", "S4 Format NG_45", "S4 燒入 此站不執行_46", "S4 燒入程式 OK_47", "S4 燒入程式 NG_48", "S4 藍芽Scan OK_49", "S4 藍芽Scan NG_50", "S4 動作完成_51", "給PLC要量電流訊號", "給PLC要量電壓訊號"]
                    n127 = call "Set OutputPLC.vi"("Address In"=20, "Array 2"=w282) -> ("Error Out"=w283:errorcluster[])  [unwired: 8 in]
                  }
                }
                n128 = global read "Main Glb.vi" "Input Registers0-99"() -> (w247:u16[])
                n129 = Select(t="OK" ("DataIn"), s=w238, f="NG" ("DataIn")) -> (s? t:f=w239:string)
                n130 = call "Red PLC InReg.vi"("length"=10, "index"=10, "Input Registers Arr"=w247) -> ("Rad In Reg"=w246:string)  [unwired: 7 in, 1 out]
                n131 = call "Cub Meaasure FGV.vi"("Action"=Table_Save."Write" ("Enum"), "Save Index"=MeasureDisplayTab."FSKscanl_315(FSK scan)", "DataIn"=w239, "SN"=w246) -> ()  [unwired: 8 in, 8 out]
                n132 = Merge Errors(w237, w236) -> (w235:errorcluster)
              }
              frame "S2" {
                # "收尋S2站條碼"
                n133 = call "Retry Num.vi"("String"=w312) -> ("Numeric"=w328:i32, "retry次數"=w325:string[])  [unwired: 9 in]
                n134 = Index Array(array=w313, index=StationCmdSelect."Command") -> (element=w306:string)
                n135 = call "ToolScanTest.vi"("error in (no error)"=w314, "VISA resource name"=refnum<visa-resource-name> "COM10") -> ("error out"=w324:errorcluster, "read string 6"=w307:string)  [unwired: 4 in, 4 out]
                "Blue Scan2 receive" <- w307
                n136 = local write "retry次數"(w325) -> ()
                n137 = call "Tool RS232 test.vi"("error in (no error)"=w314, "Cmd In"=w306, "VISA resource name"=refnum<visa-resource-name> "COM8") -> ("error out"=w331:errorcluster, "receive string"=→"S2 receive":string)  [unwired: 7 in]
                n138 = call <vilib>:"Clear Errors.vi"("error in (no error)"=w324) -> ()  [unwired: 5 in, 2 out]
                n139 = local write "CurrentCmd"(w306) -> ()
                n140 = local write "Retry"(w328) -> ()
                n141 = Unbundle By Name(w331) -> ("status"=w320:bool)
                n142 = String Length(string=w307) -> (length=w323:i32)
                n143 = Not Equal To 0?(x=w323) -> (x != 0?=w322:bool)
                n144 = Not(x=w322) -> (.not. x?=w321:bool)
                n145 = Or(x=w321, y=w320) -> (x .or. y?=w319:bool)
                n146 = Not(x=w319) -> (.not. x?=w292:bool)
                n147 = call "Auto Inspection_Status.vi"("Action"=enum16{"Initial", "Write", "Read"}."Write", "DataIn"="SCAN2", "Station"=Auto_Inspection_Station_Name2."S2Measure", "Data"=Auto_Inspection_Data_Name."CurrentAction") -> ()  [unwired: 9 in, 3 out]
                n148 = Increment(x=w311) -> (x+1=w329:i32)
                n149 = Select(t=w329, s=w319, f=w311) -> (s? t:f=w326:i32)
                n150 = Increment(x=w315) -> (x+1=w330:i32)
                n151 = Greater Or Equal?(x=w326, y=w328) -> (x >= y?=w327:bool)
                n152 = Select(t=w330, s=w292, f=w315) -> (s? t:f=w308:i32)
                n153 = case shown="True" w327 {
                  tunnel: [errorcluster {"status"=FALSE, "code"=0, "source"=""} ("error constant") errorcluster {"status"=TRUE, "code"=11505, "source"=""} ("error constant")] -> w290
                  tunnel: w326 -> [w339 _]
                  tunnel: [w339 0] -> w310
                  frame False {
                  }
                  frame True {
                  }
                }
                n154 = case shown="True" w292 {
                  tunnel: [w333 w337] -> w291
                  frame False {
                    w335 = T8[] [enum."S4 量測完成 產品NG_42"] items=["S2站PC動作中_20", "電流量測完成產品OK_21", "電流量測完成產品NG_22", "S2站Format 執行_23", "S2 Format OK_24", "S2 Format NG_25", "S2站燒入執行_26", "S2站燒入OK_27", "S2站燒入NG_28", "S2站動作完成_29", "S3 PC動作中_30", "S3 Format 此站執行_31", "S3 Format OK_32", "S3 Format NG_33", "S3 燒入程式 此站執行_34", "S3 燒入程式 OK_35", "S3 燒入程式 NG_36", "S3 備用_37", "S3 備用_38", "S3 動作完成_39", "S4 PC動作中_40", "S4 量測完成 產品正常_41", "S4 量測完成 產品NG_42", "S4 Format 此站執行_43", "S4 Format OK_44", "S4 Format NG_45", "S4 燒入 此站不執行_46", "S4 燒入程式 OK_47", "S4 燒入程式 NG_48", "S4 藍芽Scan OK_49", "S4 藍芽Scan NG_50", "S4 動作完成_51", "給PLC要量電流訊號", "給PLC要量電壓訊號"]
                    n155 = call "Set OutputPLC.vi"("Address In"=20, "Array 2"=w335) -> ("Error Out"=w333:errorcluster[])  [unwired: 8 in]
                  }
                  frame True {
                    w336 = T8[] [enum."S4 量測完成 產品正常_41"] items=["S2站PC動作中_20", "電流量測完成產品OK_21", "電流量測完成產品NG_22", "S2站Format 執行_23", "S2 Format OK_24", "S2 Format NG_25", "S2站燒入執行_26", "S2站燒入OK_27", "S2站燒入NG_28", "S2站動作完成_29", "S3 PC動作中_30", "S3 Format 此站執行_31", "S3 Format OK_32", "S3 Format NG_33", "S3 燒入程式 此站執行_34", "S3 燒入程式 OK_35", "S3 燒入程式 NG_36", "S3 備用_37", "S3 備用_38", "S3 動作完成_39", "S4 PC動作中_40", "S4 量測完成 產品正常_41", "S4 量測完成 產品NG_42", "S4 Format 此站執行_43", "S4 Format OK_44", "S4 Format NG_45", "S4 燒入 此站不執行_46", "S4 燒入程式 OK_47", "S4 燒入程式 NG_48", "S4 藍芽Scan OK_49", "S4 藍芽Scan NG_50", "S4 動作完成_51", "給PLC要量電流訊號", "給PLC要量電壓訊號"]
                    n156 = call "Set OutputPLC.vi"("Address In"=20, "Array 2"=w336) -> ("Error Out"=w337:errorcluster[])  [unwired: 8 in]
                  }
                }
                n157 = Select(t="OK" ("DataIn"), s=w292, f="NG" ("DataIn")) -> (s? t:f=w293:string)
                n158 = global read "Main Glb.vi" "Input Registers0-99"() -> (w301:u16[])
                n159 = call "Red PLC InReg.vi"("length"=10, "index"=10, "Input Registers Arr"=w301) -> ("Rad In Reg"=w300:string)  [unwired: 7 in, 1 out]
                n160 = call "Cub Meaasure FGV.vi"("Action"=Table_Save."Write" ("Enum"), "Save Index"=MeasureDisplayTab."ASKscan_433(ASK scan)", "DataIn"=w293, "SN"=w300) -> ()  [unwired: 8 in, 8 out]
                n161 = Merge Errors(w291, w290) -> (w289:errorcluster)
              }
              frame "D" {
                n162 = Index Array(array=w353, index=w350) -> (element=w352:dbl)
                n163 = Multiply(x=1000, y=w352) -> (x*y=w351:dbl)
                n164 = Wait (ms)(milliseconds to wait=w351) -> ()  [unwired: 1 out]
                n165 = call "Auto Inspection_Status.vi"("Action"=enum16{"Initial", "Write", "Read"}."Write", "DataIn"="Delay Time", "Station"=Auto_Inspection_Station_Name2."S2Measure", "Data"=Auto_Inspection_Data_Name."CurrentAction") -> ()  [unwired: 9 in, 3 out]
                n166 = Increment(x=w348) -> (x+1=w347:i32)
              }
              frame "T1" {
                (unwired) 10 ("index")
                w379 = u16 3 items=["SYSTem:VERSion?", "SYSTem:ERRor?", "*IDN?", "MEAS:CURR:DC?", "MEAS:VOLT?", "SYSTem:ERRor?"] ("Ringfor34450A")
                w378 = u16 5 items=["SYSTem:VERSion?", "SYSTem:ERRor?", "*IDN?", "MEAS:CURR:DC?", "MEAS:VOLT?", "MEAS:VOLT:DC?"] ("RingforIT8511")
                w376 = u16 1 items=["IT8511", "34450A", "WRBuff"] ("ChangeStatus")
                # "收尋S2站條碼"
                # "量電流"
                n167 = call "Retry Num.vi"("String"=w374) -> ("Numeric"=w385:i32, "retry次數"=w384:string[])  [unwired: 9 in]
                n168 = local write "retry次數"(w384) -> ()
                n169 = call "Auto Inspection_Status.vi"("Action"=enum16{"Initial", "Write", "Read"}."Write", "DataIn"="儀器34450A", "Station"=Auto_Inspection_Station_Name2."S2Measure", "Data"=Auto_Inspection_Data_Name."CurrentAction") -> ()  [unwired: 9 in, 3 out]
                n170 = local write "Retry"(w385) -> ()
                n171 = call "MTool34450A.vi"("Ringfor34450A"=w379, "RingforIT8511"=w378, "VISA resource name"=refnum<visa-resource-name> "USB0::0x2A8D::0xB318::MY59430005::INSTR", "ChangeStatus"=w376) -> ("error out"=w380:errorcluster, 1:"μA"=w359:string, 2:"μA"=→"T1 μA":dbl, "read buffer"=→"T1 buffer":string)  [unwired: 4 in]
                n172 = Unbundle By Name(w380) -> ("status"=w382:bool)
                n173 = Increment(x=w375) -> (x+1=w386:i32)
                n174 = Select(t=w386, s=w382, f=w375) -> (s? t:f=w383:i32)
                n175 = Not(x=w382) -> (.not. x?=w358:bool)
                n176 = Greater Or Equal?(x=w383, y=w385) -> (x >= y?=w381:bool)
                n177 = Increment(x=w373) -> (x+1=w387:i32)
                n178 = Select(t=w387, s=w358, f=w373) -> (s? t:f=w372:i32)
                n179 = case shown="False" w381 {
                  tunnel: [errorcluster {"status"=FALSE, "code"=0, "source"=""} ("error constant") w399] -> w356
                  tunnel: w383 -> [w397 _]
                  tunnel: [w397 0] -> w371
                  tunnel: w380 -> [_ w399]
                  frame False {
                  }
                  frame True {
                  }
                }
                n180 = Select(t=w359, s=w358, f="NG" ("DataIn")) -> (s? t:f=w360:string)
                n181 = global read "Main Glb.vi" "Input Registers0-99"() -> (w366:u16[])
                n182 = case shown="True" w358 {
                  tunnel: [w391 w394] -> w357
                  frame False {
                    w393 = T8[] [enum."電流量測完成產品NG_22"] items=["S2站PC動作中_20", "電流量測完成產品OK_21", "電流量測完成產品NG_22", "S2站Format 執行_23", "S2 Format OK_24", "S2 Format NG_25", "S2站燒入執行_26", "S2站燒入OK_27", "S2站燒入NG_28", "S2站動作完成_29", "S3 PC動作中_30", "S3 Format 此站執行_31", "S3 Format OK_32", "S3 Format NG_33", "S3 燒入程式 此站執行_34", "S3 燒入程式 OK_35", "S3 燒入程式 NG_36", "S3 備用_37", "S3 備用_38", "S3 動作完成_39", "S4 PC動作中_40", "S4 量測完成 產品正常_41", "S4 量測完成 產品NG_42", "S4 Format 此站執行_43", "S4 Format OK_44", "S4 Format NG_45", "S4 燒入 此站不執行_46", "S4 燒入程式 OK_47", "S4 燒入程式 NG_48", "S4 藍芽Scan OK_49", "S4 藍芽Scan NG_50", "S4 動作完成_51", "給PLC要量電流訊號", "給PLC要量電壓訊號"]
                    n183 = call "Set OutputPLC.vi"("Address In"=20, "Array 2"=w393) -> ("Error Out"=w391:errorcluster[])  [unwired: 8 in]
                  }
                  frame True {
                    w395 = T8[] [enum."電流量測完成產品OK_21"] items=["S2站PC動作中_20", "電流量測完成產品OK_21", "電流量測完成產品NG_22", "S2站Format 執行_23", "S2 Format OK_24", "S2 Format NG_25", "S2站燒入執行_26", "S2站燒入OK_27", "S2站燒入NG_28", "S2站動作完成_29", "S3 PC動作中_30", "S3 Format 此站執行_31", "S3 Format OK_32", "S3 Format NG_33", "S3 燒入程式 此站執行_34", "S3 燒入程式 OK_35", "S3 燒入程式 NG_36", "S3 備用_37", "S3 備用_38", "S3 動作完成_39", "S4 PC動作中_40", "S4 量測完成 產品正常_41", "S4 量測完成 產品NG_42", "S4 Format 此站執行_43", "S4 Format OK_44", "S4 Format NG_45", "S4 燒入 此站不執行_46", "S4 燒入程式 OK_47", "S4 燒入程式 NG_48", "S4 藍芽Scan OK_49", "S4 藍芽Scan NG_50", "S4 動作完成_51", "給PLC要量電流訊號", "給PLC要量電壓訊號"]
                    n184 = call "Set OutputPLC.vi"("Address In"=20, "Array 2"=w395) -> ("Error Out"=w394:errorcluster[])  [unwired: 8 in]
                  }
                }
                n185 = call "Red PLC InReg.vi"("length"=10, "Input Registers Arr"=w366) -> ("Rad In Reg"=w365:string)  [unwired: 8 in, 1 out]
                n186 = call "Cub Meaasure FGV.vi"("Action"=Table_Save."Write" ("Enum"), "Save Index"=MeasureDisplayTab."耗電流 uA(電流表)", "DataIn"=w360, "SN"=w365) -> ()  [unwired: 8 in, 8 out]
                n187 = Merge Errors(w357, w356) -> (w355:errorcluster)
              }
              frame "T2" {
                w428 = u16 3 items=["SYSTem:VERSion?", "SYSTem:ERRor?", "*IDN?", "MEAS:CURR:DC?", "MEAS:VOLT?", "SYSTem:ERRor?"] ("Ringfor34450A")
                w427 = u16 5 items=["SYSTem:VERSion?", "SYSTem:ERRor?", "*IDN?", "MEAS:CURR:DC?", "MEAS:VOLT?", "MEAS:VOLT:DC?"] ("RingforIT8511")
                w425 = u16 0 items=["IT8511", "34450A", "WRBuff"] ("ChangeStatus")
                # "收尋S2站條碼"
                # "量電壓"
                n188 = call "Auto Inspection_Status.vi"("Action"=enum16{"Initial", "Write", "Read"}."Write", "DataIn"="IT8511", "Station"=Auto_Inspection_Station_Name2."S2Measure", "Data"=Auto_Inspection_Data_Name."CurrentAction") -> ()  [unwired: 9 in, 3 out]
                n189 = call "Retry Num.vi"("String"=w419) -> ("Numeric"=w434:i32, "retry次數"=w433:string[])  [unwired: 9 in]
                n190 = local write "retry次數"(w433) -> ()
                n191 = local write "Retry"(w434) -> ()
                n192 = call "MTool34450A.vi"("Ringfor34450A"=w428, "RingforIT8511"=w427, "VISA resource name"=refnum<visa-resource-name> "COM11", "ChangeStatus"=w425) -> ("error out"=w430:errorcluster, "μA"=→"T2 μA":dbl, "read buffer"=w406:string)  [unwired: 4 in, 1 out]
                "T2 buffer" <- w406
                n193 = Unbundle By Name(w430) -> ("status"=w404:bool)
                n194 = Increment(x=w420) -> (x+1=w429:i32)
                n195 = Not(x=w404) -> (.not. x?=w405:bool)
                n196 = Select(t=w429, s=w404, f=w429) -> (s? t:f=w432:i32)
                n197 = Greater Or Equal?(x=w432, y=w434) -> (x >= y?=w431:bool)
                n198 = Increment(x=w421) -> (x+1=w435:i32)
                n199 = Select(t=w406, s=w405, f="NG" ("DataIn")) -> (s? t:f=w407:string)
                n200 = global read "Main Glb.vi" "Input Registers0-99"() -> (w414:u16[])
                n201 = Select(t=w435, s=w405, f=w421) -> (s? t:f=w422:i32)
                n202 = case shown="False" w431 {
                  tunnel: [errorcluster {"status"=FALSE, "code"=0, "source"=""} ("error constant") w445] -> w402
                  tunnel: w432 -> [w443 _]
                  tunnel: [w443 0] -> w424
                  tunnel: w430 -> [_ w445]
                  frame False {
                  }
                  frame True {
                  }
                }
                n203 = case shown="False" w404 {
                  tunnel: [w437 w440] -> w403
                  frame False {
                    w439 = T8[] [enum."S4 量測完成 產品NG_42"] items=["S2站PC動作中_20", "電流量測完成產品OK_21", "電流量測完成產品NG_22", "S2站Format 執行_23", "S2 Format OK_24", "S2 Format NG_25", "S2站燒入執行_26", "S2站燒入OK_27", "S2站燒入NG_28", "S2站動作完成_29", "S3 PC動作中_30", "S3 Format 此站執行_31", "S3 Format OK_32", "S3 Format NG_33", "S3 燒入程式 此站執行_34", "S3 燒入程式 OK_35", "S3 燒入程式 NG_36", "S3 備用_37", "S3 備用_38", "S3 動作完成_39", "S4 PC動作中_40", "S4 量測完成 產品正常_41", "S4 量測完成 產品NG_42", "S4 Format 此站執行_43", "S4 Format OK_44", "S4 Format NG_45", "S4 燒入 此站不執行_46", "S4 燒入程式 OK_47", "S4 燒入程式 NG_48", "S4 藍芽Scan OK_49", "S4 藍芽Scan NG_50", "S4 動作完成_51", "給PLC要量電流訊號", "給PLC要量電壓訊號"]
                    n204 = call "Set OutputPLC.vi"("Address In"=20, "Array 2"=w439) -> ("Error Out"=w437:errorcluster[])  [unwired: 8 in]
                  }
                  frame True {
                    w441 = T8[] [enum."S4 量測完成 產品正常_41"] items=["S2站PC動作中_20", "電流量測完成產品OK_21", "電流量測完成產品NG_22", "S2站Format 執行_23", "S2 Format OK_24", "S2 Format NG_25", "S2站燒入執行_26", "S2站燒入OK_27", "S2站燒入NG_28", "S2站動作完成_29", "S3 PC動作中_30", "S3 Format 此站執行_31", "S3 Format OK_32", "S3 Format NG_33", "S3 燒入程式 此站執行_34", "S3 燒入程式 OK_35", "S3 燒入程式 NG_36", "S3 備用_37", "S3 備用_38", "S3 動作完成_39", "S4 PC動作中_40", "S4 量測完成 產品正常_41", "S4 量測完成 產品NG_42", "S4 Format 此站執行_43", "S4 Format OK_44", "S4 Format NG_45", "S4 燒入 此站不執行_46", "S4 燒入程式 OK_47", "S4 燒入程式 NG_48", "S4 藍芽Scan OK_49", "S4 藍芽Scan NG_50", "S4 動作完成_51", "給PLC要量電流訊號", "給PLC要量電壓訊號"]
                    n205 = call "Set OutputPLC.vi"("Address In"=20, "Array 2"=w441) -> ("Error Out"=w440:errorcluster[])  [unwired: 8 in]
                  }
                }
                n206 = call "Red PLC InReg.vi"("length"=10, "index"=10, "Input Registers Arr"=w414) -> ("Rad In Reg"=w413:string)  [unwired: 7 in, 1 out]
                n207 = call "Cub Meaasure FGV.vi"("Action"=Table_Save."Write" ("Enum"), "Save Index"=MeasureDisplayTab."電池負載電壓", "DataIn"=w407, "SN"=w413) -> ()  [unwired: 8 in, 8 out]
                n208 = Merge Errors(w403, w402) -> (w401:errorcluster)
              }
            }
          }
          frame True {
            w447 = TRUE
            "Boolean" <- w447
          }
        }
        n209 = property class="DigNum (strict)"(reference=w62, "Value"=w61) -> ()  [unwired: 1 in, 2 out]
        n210 = Compound Arithmetic op=OR(w59, w66, "stop") -> (w65:bool)
      }
    }
    frame Enabled {
    }
  }
  n211 = disable-structure shown="Disabled" {
    frame Disabled {
      n212 = while {
        tunnel: cluster{"Table Control":string[][]}[] [{"Table Control"=[]}] ("Array 2") -> [w455]
        shift-right: [w454] -> w448
        shift-left: _ -> [w452]
        stop <- TRUE stop-if-true
        n213 = case shown="\"Add\"" "Enum" {
          tunnel: w455 -> [w457 _ _ _ _ _]
          tunnel: [w457 w461 w466 w491 w513 w520] -> w454
          tunnel: "Table Control 3" -> [_ w459 w468 w482 _ _]
          tunnel: w452 -> [_ w458 w463 w489 w512 w520]
          tunnel: "SN" -> [_ _ w462 w488 w511 _]
          frame "initial", Default {
          }
          frame "Add" {
            n214 = Bundle("Table Control 3"=w459) -> (w460:cluster{"Table Control 3":string[][]})  [unwired: 1 in]
            n215 = Build Array (concatenate)(w458, w460) -> (w461:cluster{"Table Control 3":string[][]}[])
            n216 = Bundle() -> ()  [unwired: 2 in, 1 out]
          }
          frame "Write" {
            n217 = for {
              tunnel: w463 -> [w476] mode=indexing
              tunnel: [w472] -> w471 mode=indexing
              n218 = Unbundle By Name(w476) -> ("Table Control 3"=w475:string[][])
              n219 = Index Array(array=w475, index (row)=0 ("disabled index (col)"), index (col)=1 ("disabled index (col)")) -> (element=w472:string)
            }
            n220 = Search 1D Array(1D array=w471, element=w462) -> (index of element=w467:i32)  [unwired: 1 in]
            n221 = Index Array(array=w463, index=w467) -> (element=w470:cluster{"Table Control 3":string[][]})
            n222 = Unbundle By Name(w470) -> ("Table Control 3"=w469:string[][])
            n223 = Build Array (concatenate)(w469, w468) -> (w465:string[][])
            n224 = Bundle(w465) -> (w464:cluster{string[][]})  [unwired: 1 in]
            n225 = Replace Array Subset(array=w463, new element=w464, index=w467) -> (w466:cluster{"Table Control 3":string[][]}[])
          }
          frame "Replace" {
            n226 = for {
              tunnel: w489 -> [w505] mode=indexing
              tunnel: [w501] -> w493 mode=indexing
              n227 = Unbundle By Name(w505) -> ("Table Control 3"=w504:string[][])
              n228 = Index Array(array=w504, index (row)=0 ("disabled index (col)"), index (col)=1 ("disabled index (col)")) -> (element=w501:string)
            }
            n229 = Search 1D Array(1D array=w493, element=w488) -> (index of element=w486:i32)  [unwired: 1 in]
            n230 = Index Array(array=w489, index=w486) -> (element=w492:cluster{"Table Control 3":string[][]})
            n231 = Unbundle By Name(w492) -> ("Table Control 3"=w479:string[][])
            n232 = Array Size(array=w482) -> (size(s)=w484:i32[])
            n233 = Index Array(array=w482, index (col)=1 ("disabled index (col)")) -> (element=w480:string[])  [unwired: 1 in]
            n234 = Index Array(array=w484) -> (element #1=w483:i32)  [unwired: 2 in, 1 out]
            n235 = Array Size(array=w479) -> (size(s)=w485:i32[])
            n236 = Index Array(array=w485) -> (element #1=w478:i32)  [unwired: 2 in, 1 out]
            n237 = Subtract(x=w478, y=w483) -> (x-y=w477:i32)
            n238 = for {
              shift-right: [w500] -> w487
              shift-left: w479 -> [w499]
              tunnel: w477 -> [w496]
              tunnel: w480 -> [w495] mode=indexing
              i -> [w497]
              n239 = Add(x=w496, y=w497) -> (x+y=w494:i32)
              n240 = Replace Array Subset(array=w499, new element=w495, index (row)=w494, index (col)=1 ("disabled index (col)")) -> (w500:string[][])
            }
            n241 = Bundle("Table Control 3"=w487) -> (w490:cluster{"Table Control 3":string[][]})  [unwired: 1 in]
            n242 = Replace Array Subset(array=w489, new element=w490, index=w486) -> (w491:cluster{"Table Control 3":string[][]}[])
          }
          frame "Delete" {
            n243 = for {
              tunnel: w512 -> [w519] mode=indexing
              tunnel: [w515] -> w514 mode=indexing
              n244 = Unbundle By Name(w519) -> ("Table Control 3"=w518:string[][])
              n245 = Index Array(array=w518, index (row)=0 ("disabled index (col)"), index (col)=1 ("disabled index (col)")) -> (element=w515:string)
            }
            n246 = Search 1D Array(1D array=w514, element=w511) -> (index of element=w510:i32)  [unwired: 1 in]
            n247 = Index Array(array=w512, index=w510) -> ()  [unwired: 1 out]
            n248 = Delete From Array(array=w512, length=1, index=w510) -> (deleted portion=w508:cluster{"Table Control 3":string[][]}[], array with subset deleted=w513:cluster{"Table Control 3":string[][]}[])
            n249 = Index Array(array=w508) -> (element=w507:cluster{"Table Control 3":string[][]})  [unwired: 1 in]
            n250 = Unbundle By Name(w507) -> ("Table Control 3"=→"LOG":string[][])
          }
          frame "REad" {
          }
        }
      }
      "Array 3" <- w448
    }
    frame Enabled {
    }
  }
  n251 = disable-structure shown="Disabled" {
    frame Disabled {
      n252 = call "Save Table Test.vi"() -> ()  [unwired: 10 in, 2 out]
    }
    frame Enabled {
    }
  }
